vi "Configure Build Types.vi"(7 "Build Types":T1[](array[typedef]), 8 "error in (no error)":errorcluster, 11 "CD Build Tools in":refnum<class "Project Build Tools.lvclass">) -> (0 "error out":errorcluster, 3 "CD Build Tools out":refnum<class "Project Build Tools.lvclass">)   [LabVIEW 2019, in "Project Build Tools.lvclass"]
uses:
  Project Build Tools.lvclass
  TypeDefs/Configure Build Types.ctl
  Project Build Tools.lvclass/Project Build Tools.ctl
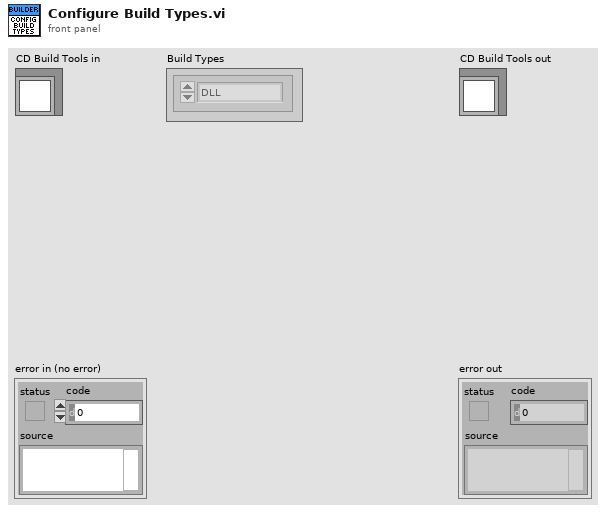
[diagram p1: front panel]
types:
  T1 = typedef "Project Build Tools.lvclass/Configure Build Types.ctl" = enum16{"DLL", "Packed Library", "Installer", "Source Distribution", "EXE"}
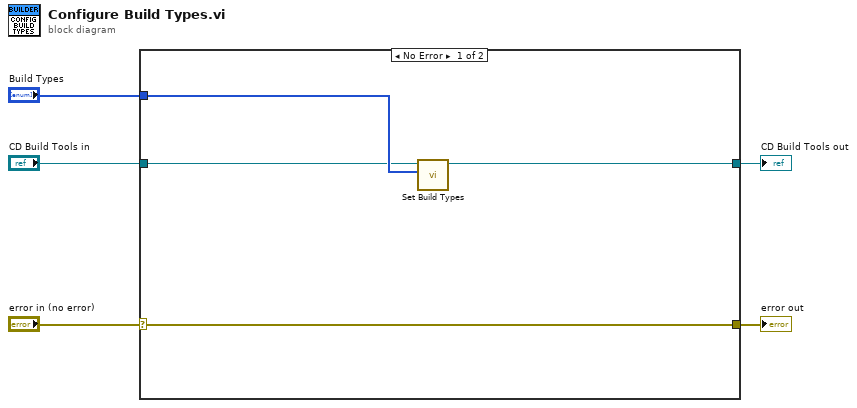
[diagram p0: block diagram]
diagram:
  n1 = case shown="No Error" "error in (no error)" {
    selector: "error in (no error)" -> [w9 w11]
    tunnel: [w9 w11] -> w4
    tunnel: [w7 w10] -> w2
    tunnel: "CD Build Tools in" -> [w6 w10]
    tunnel: "Build Types" -> [w8 _]
    frame No Error {
      n2 = call "Set Build Types.vi"("Build Types"=w8, "CD Build Tools in"=w6) -> ("CD Build Tools out"=w7:refnum<class "Project Build Tools.lvclass">)  [unwired: 9 in]
    }
    frame Error {
    }
  }
  "error out" <- w4
  "CD Build Tools out" <- w2
